vi "8.4 N-channel Acquisition Data Types.vi"() -> ()   [LabVIEW 2019]
uses:
  <vilib>/DAQmx/read.llb/DAQmx Read (Analog 1D DBL NChan 1Samp).vi
  <vilib>/DAQmx/create/channels.llb/DAQmx Create Channel (AI-Voltage-Basic).vi
  <vilib>/DAQmx/configure/timing.llb/DAQmx Timing (Sample Clock).vi
  <vilib>/DAQmx/miscellaneous.llb/DAQmx Fill In Error Info.vi
  <resource>/objmgr/daqmx.rc
panel:
  out "Waveform Chart":T1(graph)
  in  "task in":refnum<k21>
  out "1D Numeric Output":dbl[](array[numeric])
  in  "Stop":bool
  out "Actual Sample Rate (Hz)":dbl
  in  "Configuration Control":T2={"number of samples"=-1, "Minimum Value"=-1.0, "Maximum Value"=-1.0, "physical channels"="Multi_I-O/ai0", "Desired Sample Rate (Hz)"=-1.0, "sample mode"=10178} {"sample mode" items=["Finite Samples"=10178, "Continuous Samples"=10123, "Hardware Timed Single Point"=12522]}
  # "Full DAQmx API"
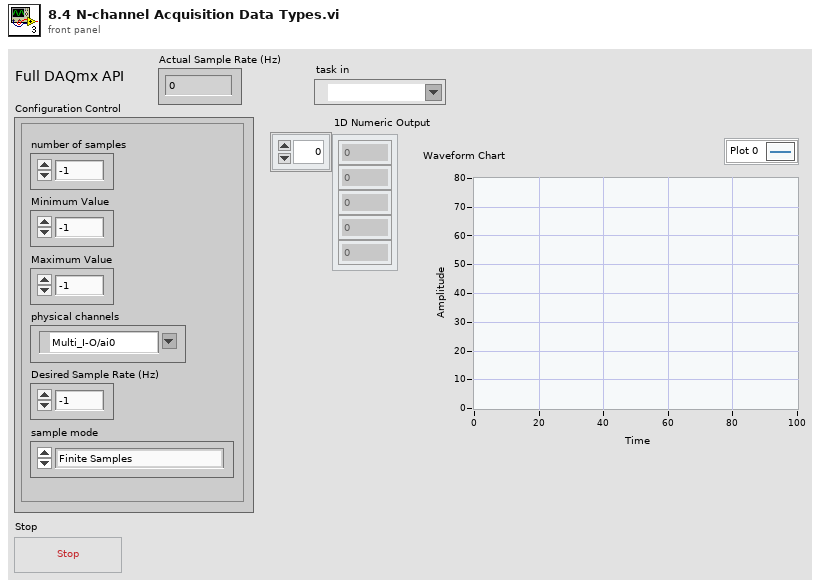
[diagram p1: front panel]
types:
  T1 = cluster{"data[0]":dbl, "data[1]":dbl, "data[2]":dbl, "data[3]":dbl, "data[4]":dbl, "data[5]":dbl, "data[6]":dbl, "data[7]":dbl, "data[8]":dbl}
  T2 = cluster{"number of samples":i32, "Minimum Value":dbl, "Maximum Value":dbl, "physical channels":tag, "Desired Sample Rate (Hz)":dbl, "sample mode":i32}
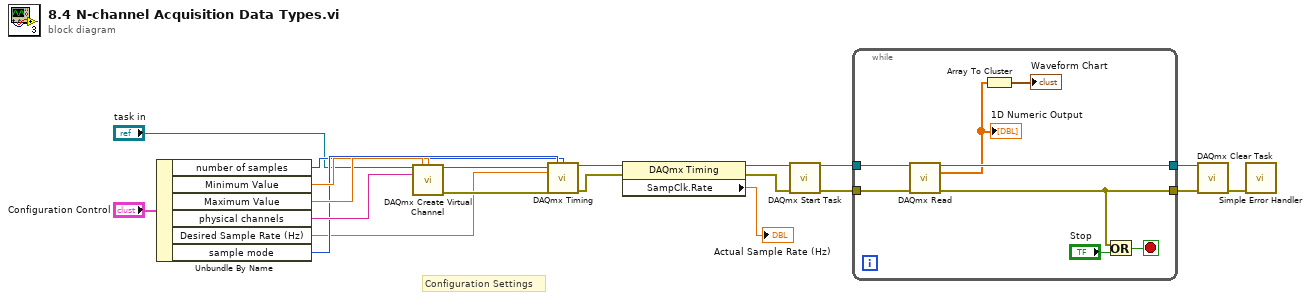
[diagram p0: block diagram]
diagram:
  # "Configuration Settings"
  n1 = Unbundle By Name("Configuration Control") -> ("number of samples"=w5:i32, "Minimum Value"=w16:dbl, "Maximum Value"=w17:dbl, "physical channels"=w15:tag, "Desired Sample Rate (Hz)"=w13:dbl, "sample mode"=w14:i32)
  n2 = call-poly <vilib>:"DAQmx Create Virtual Channel.vi"("task in"="task in", "maximum value"=w17, "minimum value"=w16, "physical channels"=w15) -> ("task out"=w20:refnum<k21>, "error out"=w19:errorcluster)  [unwired: 10 in]
  n3 = call-poly <vilib>:"DAQmx Timing.vi"("task/channels in"=w20, "sample mode"=w14, "samples per channel"=w5, "rate"=w13, "error in"=w19) -> ("task out"=w11:refnum<k21>, "error out"=w12:errorcluster)  [unwired: 9 in]
  n4 = property class="DAQmx Timing"(reference=w11, error in=w12) -> (reference out=w8:refnum<k21>, error out=w7:errorcluster, "SampClk.Rate"=→"Actual Sample Rate (Hz)":dbl)
  n5 = call <vilib>:"DAQmx Start Task.vi"("task/channels in"=w8, "error in"=w7) -> ("task out"=w9:refnum<k21>, "error out"=w6:errorcluster)  [unwired: 12 in]
  n6 = while {
    tunnel: w9 -> [w28]
    tunnel: w6 -> [w27]
    tunnel: [w26] -> w3
    tunnel: [w21] -> w2
    stop <- w22 stop-if-true
    n7 = call-poly <vilib>:"DAQmx Read.vi"("task/channels in"=w28, "error in"=w27) -> ("task out"=w26:refnum<k21>, "data"=w25:dbl[], "error out"=w21:errorcluster)  [unwired: 11 in]
    "1D Numeric Output" <- w25
    n8 = Array To Cluster(array=w25) -> (cluster=→"Waveform Chart":T1)
    n9 = Or(x=w21, y="Stop") -> (x .or. y?=w22:bool)
  }
  n10 = call <vilib>:"DAQmx Clear Task.vi"("task in"=w3, "error in"=w2) -> ("error out"=w4:errorcluster)  [unwired: 13 in]
  n11 = call <vilib>:"Simple Error Handler.vi"("error in (no error)"=w4) -> ()  [unwired: 4 in, 5 out]
